vi "X Array Index to Range.vi"(1 "X Range (points)":i32=1, 2 "X-array":dbl[](array[numeric])) -> (0 "X Range (data)":dbl)   [LabVIEW 2016, in "xy_utilities.lvlib"]
uses:
  xy_utilities.lvlib
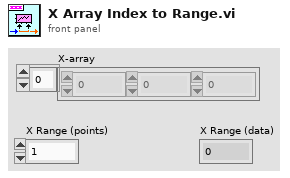
[diagram p1: front panel]
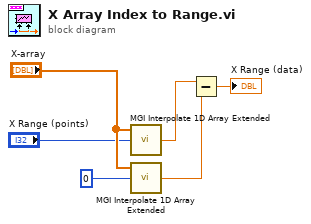
[diagram p0: block diagram]
diagram:
  n1 = call <userlib>:"MGI Interpolate 1D Array Extended.vi"("Fractional X"="X Range (points)", "Y Value[]"="X-array") -> ("ExtendedY"=w1:dbl)  [unwired: 1 in]
  n2 = call <userlib>:"MGI Interpolate 1D Array Extended.vi"("Fractional X"=0 ("index"), "Y Value[]"="X-array") -> ("ExtendedY"=w2:dbl)  [unwired: 1 in]
  n3 = Subtract(x=w1, y=w2) -> (x-y=→"X Range (data)":dbl)
